vi "int16ToFuzzyMap.vi"(8 "Input Registers":u16[](array[numeric])) -> (0 "Table Control":string[][](table))   [LabVIEW 2016]
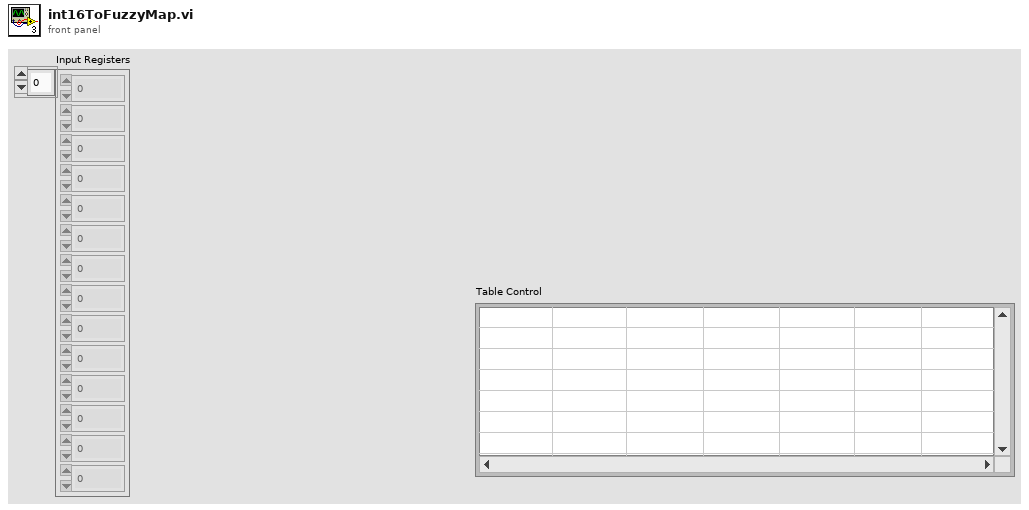
[diagram p1: front panel]
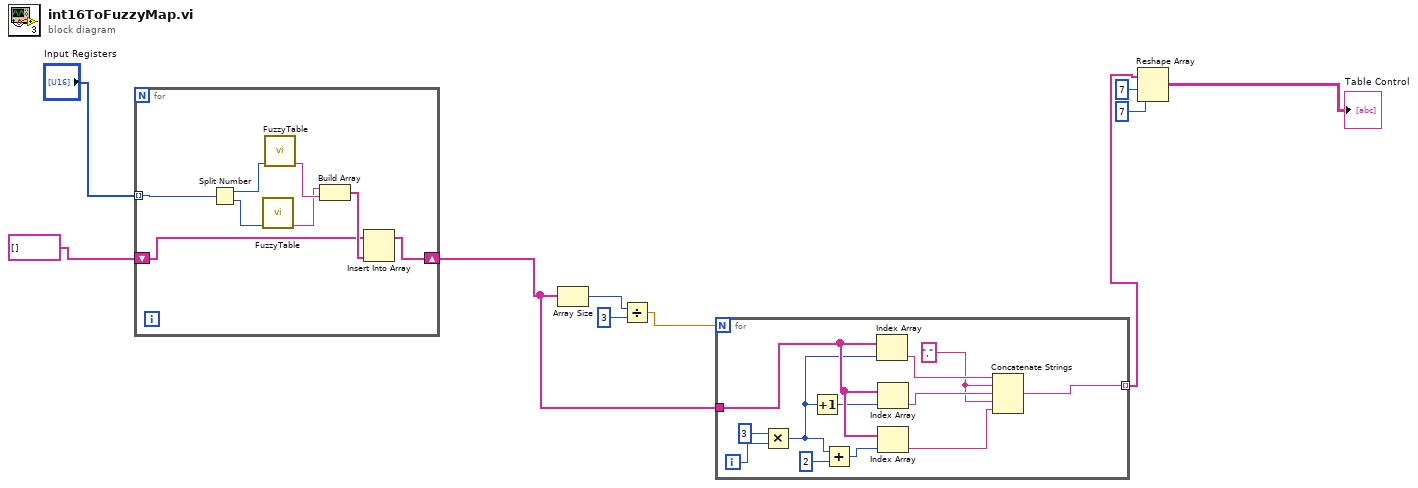
[diagram p0: block diagram]
diagram:
  n1 = for {
    tunnel: "Input Registers" -> [w18] mode=indexing
    shift-right: [w11] -> w5
    shift-left: string[] [] ("array") -> [w12]
    n2 = Split Number(x=w18) -> (hi(x)=w17:u8, lo(x)=w15:u8)
    n3 = call "FuzzyTable.vi"("Numeric"=w15) -> ("String"=w14:string)  [unwired: 10 in]
    n4 = call "FuzzyTable.vi"("Numeric"=w17) -> ("String"=w16:string)  [unwired: 10 in]
    n5 = Build Array(w14, w16) -> (w13:string[])
    n6 = Insert Into Array(array=w12, new element=w13) -> (w11:string[])  [unwired: 1 in]
  }
  n7 = Array Size(array=w5) -> (size(s)=w8:i32)
  n8 = Divide(x=w8, y=3) -> (x/y=w6:dbl)
  n9 = for {
    N: w6 -> [_]
    tunnel: w5 -> [w30]
    tunnel: [w21] -> w2 mode=indexing
    i -> [w29]
    w19 = "," ("string")
    n10 = Multiply(x=3, y=w29) -> (x*y=w24:i32)
    n11 = Increment(x=w24) -> (x+1=w25:i32)
    n12 = Add(x=w24, y=2) -> (x+y=w27:i32)
    n13 = Index Array(array=w30, index=w24) -> (element=w23:string)
    n14 = Index Array(array=w30, index=w25) -> (element=w20:string)
    n15 = Index Array(array=w30, index=w27) -> (element=w22:string)
    n16 = Concatenate Strings(w23, w19, w20, w19, w22) -> (w21:string)
  }
  n17 = Reshape Array(w2, 7 ("dimension size"), 7 ("dimension size")) -> (→"Table Control":string[][])
